vi "WriteIndicatorsToNT.vi"   [LabVIEW 2019]
uses:
  Globals/Sensor_Values.vi
  <vilib>/Rock Robotics/Network Tables/NT Write Number.vi
  <vilib>/Rock Robotics/Network Tables/NT Write Boolean.vi
  Globals/Dash_Globals.vi
  <vilib>/Rock Robotics/Network Tables/NT Read String.vi
  <vilib>/Rock Robotics/Network Tables/NT Write String.vi
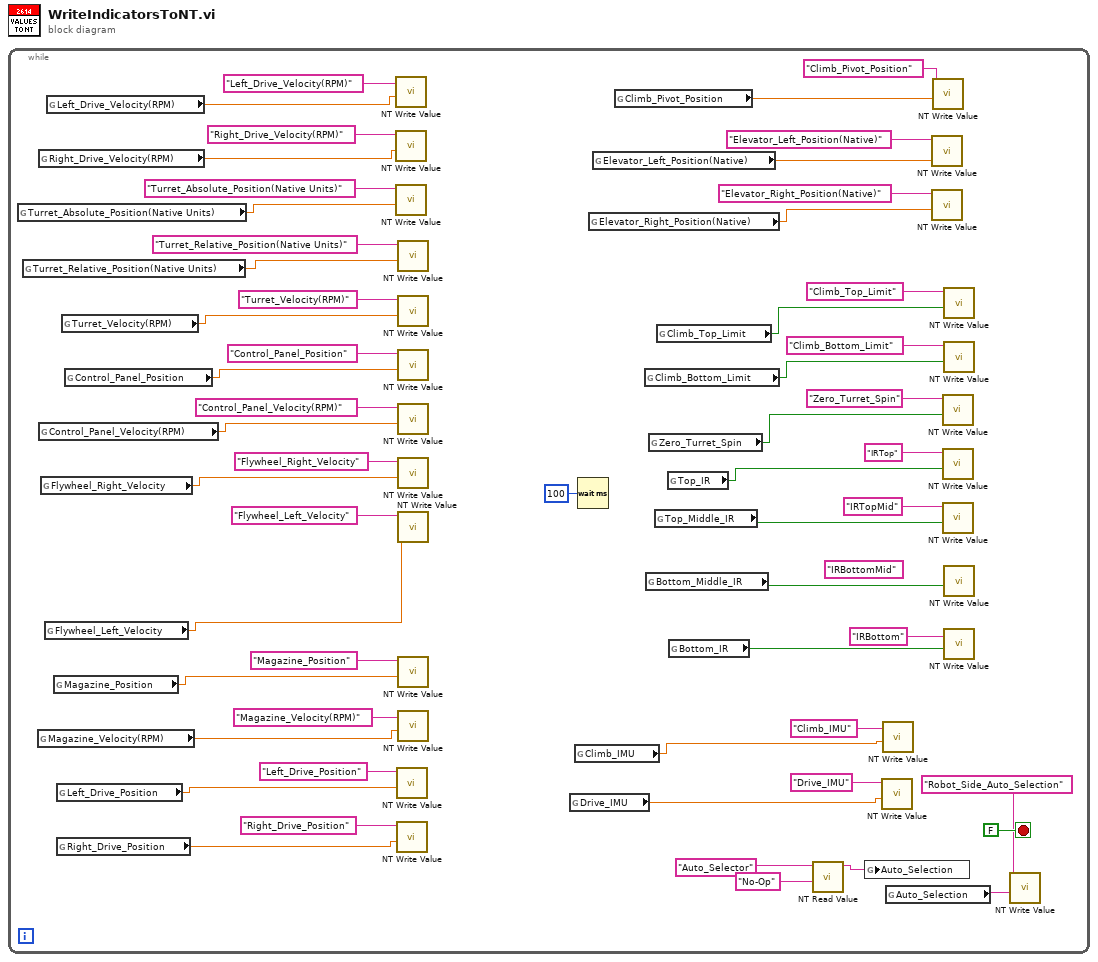
[diagram p0: block diagram]
diagram:
  n1 = while {
    stop <- FALSE stop-if-true
    (unwired) "IRBottomMid" ("Name")
    n2 = global read "Sensor_Values.vi" "Turret_Absolute_Position(Native Units)"() -> (w15:dbl)
    n3 = global read "Sensor_Values.vi" "Turret_Relative_Position(Native Units)"() -> (w14:dbl)
    n4 = global read "Sensor_Values.vi" "Magazine_Velocity(RPM)"() -> (w45:dbl)
    n5 = global read "Sensor_Values.vi" "Right_Drive_Velocity(RPM)"() -> (w46:dbl)
    n6 = global read "Sensor_Values.vi" "Control_Panel_Velocity(RPM)"() -> (w41:dbl)
    n7 = global read "Sensor_Values.vi" "Flywheel_Right_Velocity"() -> (w42:dbl)
    n8 = global read "Sensor_Values.vi" "Flywheel_Left_Velocity"() -> (w43:dbl)
    n9 = global read "Sensor_Values.vi" "Left_Drive_Velocity(RPM)"() -> (w12:dbl)
    n10 = global read "Sensor_Values.vi" "Magazine_Position"() -> (w44:dbl)
    n11 = global read "Sensor_Values.vi" "Left_Drive_Position"() -> (w37:dbl)
    n12 = global read "Sensor_Values.vi" "Right_Drive_Position"() -> (w36:dbl)
    n13 = global read "Sensor_Values.vi" "Turret_Velocity(RPM)"() -> (w39:dbl)
    n14 = global read "Sensor_Values.vi" "Control_Panel_Position"() -> (w40:dbl)
    n15 = call-poly <vilib>:"NT Write Value.vi"("Numeric"=w12, "Name"="Left_Drive_Velocity(RPM)") -> ()  [unwired: 9 in, 1 out]
    n16 = call-poly <vilib>:"NT Write Value.vi"("Numeric"=w46, "Name"="Right_Drive_Velocity(RPM)") -> ()  [unwired: 9 in, 1 out]
    n17 = call-poly <vilib>:"NT Write Value.vi"("Numeric"=w15, "Name"="Turret_Absolute_Position(Native Units)") -> ()  [unwired: 9 in, 1 out]
    n18 = call-poly <vilib>:"NT Write Value.vi"("Numeric"=w37, "Name"="Left_Drive_Position") -> ()  [unwired: 9 in, 1 out]
    n19 = call-poly <vilib>:"NT Write Value.vi"("Numeric"=w36, "Name"="Right_Drive_Position") -> ()  [unwired: 9 in, 1 out]
    n20 = call-poly <vilib>:"NT Write Value.vi"("Numeric"=w14, "Name"="Turret_Relative_Position(Native Units)") -> ()  [unwired: 9 in, 1 out]
    n21 = call-poly <vilib>:"NT Write Value.vi"("Numeric"=w39, "Name"="Turret_Velocity(RPM)") -> ()  [unwired: 9 in, 1 out]
    n22 = call-poly <vilib>:"NT Write Value.vi"("Numeric"=w40, "Name"="Control_Panel_Position") -> ()  [unwired: 9 in, 1 out]
    n23 = call-poly <vilib>:"NT Write Value.vi"("Numeric"=w41, "Name"="Control_Panel_Velocity(RPM)") -> ()  [unwired: 9 in, 1 out]
    n24 = call-poly <vilib>:"NT Write Value.vi"("Numeric"=w42, "Name"="Flywheel_Right_Velocity") -> ()  [unwired: 9 in, 1 out]
    n25 = call-poly <vilib>:"NT Write Value.vi"("Numeric"=w43, "Name"="Flywheel_Left_Velocity") -> ()  [unwired: 9 in, 1 out]
    n26 = call-poly <vilib>:"NT Write Value.vi"("Numeric"=w44, "Name"="Magazine_Position") -> ()  [unwired: 9 in, 1 out]
    n27 = call-poly <vilib>:"NT Write Value.vi"("Numeric"=w45, "Name"="Magazine_Velocity(RPM)") -> ()  [unwired: 9 in, 1 out]
    n28 = global read "Sensor_Values.vi" "Drive_IMU"() -> (w7:dbl)
    n29 = global read "Sensor_Values.vi" "Climb_IMU"() -> (w8:dbl)
    n30 = Wait (ms)(milliseconds to wait=u32 100) -> ()  [unwired: 1 out]
    n31 = global read "Sensor_Values.vi" "Elevator_Right_Position(Native)"() -> (w20:dbl)
    n32 = global read "Sensor_Values.vi" "Elevator_Left_Position(Native)"() -> (w22:dbl)
    n33 = global read "Sensor_Values.vi" "Climb_Pivot_Position"() -> (w24:dbl)
    n34 = global read "Sensor_Values.vi" "Climb_Bottom_Limit"() -> (w16:bool)
    n35 = global read "Sensor_Values.vi" "Bottom_Middle_IR"() -> (w1:bool)
    n36 = global read "Sensor_Values.vi" "Zero_Turret_Spin"() -> (w11:bool)
    n37 = global read "Sensor_Values.vi" "Top_Middle_IR"() -> (w33:bool)
    n38 = global read "Sensor_Values.vi" "Climb_Top_Limit"() -> (w17:bool)
    n39 = global read "Sensor_Values.vi" "Top_IR"() -> (w34:bool)
    n40 = global read "Sensor_Values.vi" "Bottom_IR"() -> (w32:bool)
    n41 = call-poly <vilib>:"NT Read Value.vi"("Default Value"="No-Op", "Name"="Auto_Selector") -> ("String"=w3:string)  [unwired: 8 in, 1 out]
    n42 = global write "Dash_Globals.vi" "Auto_Selection"(w3) -> ()
    n43 = call-poly <vilib>:"NT Write Value.vi"("Numeric"=w7, "Name"="Drive_IMU") -> ()  [unwired: 9 in, 1 out]
    n44 = call-poly <vilib>:"NT Write Value.vi"("Numeric"=w8, "Name"="Climb_IMU") -> ()  [unwired: 9 in, 1 out]
    n45 = global read "Dash_Globals.vi" "Auto_Selection"() -> (w2:string)
    n46 = call-poly <vilib>:"NT Write Value.vi"("Numeric"=w22, "Name"="Elevator_Left_Position(Native)") -> ()  [unwired: 9 in, 1 out]
    n47 = call-poly <vilib>:"NT Write Value.vi"("Numeric"=w20, "Name"="Elevator_Right_Position(Native)") -> ()  [unwired: 9 in, 1 out]
    n48 = call-poly <vilib>:"NT Write Value.vi"("Numeric"=w24, "Name"="Climb_Pivot_Position") -> ()  [unwired: 9 in, 1 out]
    n49 = call-poly <vilib>:"NT Write Value.vi"("Boolean"=w11, "Name"="Zero_Turret_Spin") -> ()  [unwired: 9 in, 1 out]
    n50 = call-poly <vilib>:"NT Write Value.vi"("Boolean"=w34, "Name"="IRTop") -> ()  [unwired: 9 in, 1 out]
    n51 = call-poly <vilib>:"NT Write Value.vi"("Boolean"=w33, "Name"="IRTopMid") -> ()  [unwired: 9 in, 1 out]
    n52 = call-poly <vilib>:"NT Write Value.vi"("Boolean"=w17, "Name"="Climb_Top_Limit") -> ()  [unwired: 9 in, 1 out]
    n53 = call-poly <vilib>:"NT Write Value.vi"("Boolean"=w16, "Name"="Climb_Bottom_Limit") -> ()  [unwired: 9 in, 1 out]
    n54 = call-poly <vilib>:"NT Write Value.vi"("Boolean"=w1) -> ()  [unwired: 10 in, 1 out]
    n55 = call-poly <vilib>:"NT Write Value.vi"("Boolean"=w32, "Name"="IRBottom") -> ()  [unwired: 9 in, 1 out]
    n56 = call-poly <vilib>:"NT Write Value.vi"("String"=w2, "Name"="Robot_Side_Auto_Selection") -> ()  [unwired: 9 in, 1 out]
  }
